vi "checkRowColor.vi"(8 "error in (no error)":errorcluster, 9 "add/delete":bool, 10 "Table in":refnum<vi>, 11 "reference in":refnum<class "Project Panels.lvclass">) -> (0 "error out":errorcluster, 3 "reference out":refnum<class "Project Panels.lvclass">)   [LabVIEW 2014, in "Project Panels.lvclass"]
uses:
  Project Panels.lvclass
  SYS/Notification Controller_class/Notification Controller.lvclass
  APP/trackingNotification_class/trackingNotification.lvclass
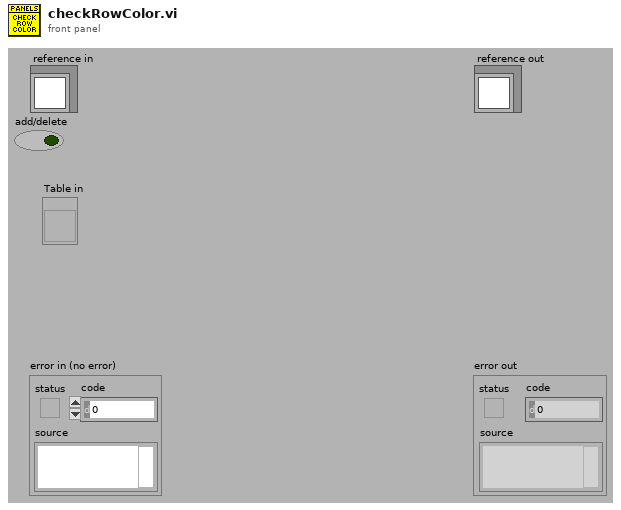
[diagram p1: front panel]
types:
  T1 = typedef "Project Panels.lvclass/ObjectAttributesRef.ctl" = refnum<data-value>
  T2 = typedef "Project Panels.lvclass/ObjectAttributes.ctl" = cluster{"MyAttribute":dbl, "device_controller_ref":refnum<class "Devices Controller.lvclass">, "file_controller_ref":refnum<class "File Controller.lvclass">, "item_controller_ref":refnum<class "Items Controller.lvclass">, "item_tables":cluster{"checkIN":string[][], "checkOUT":string[][], "storage":string[][]}, "quickbook_table":cluster{"notes":string[][]}, "notification_controller_ref":refnum<class "Notification Controller.lvclass">, "partstracking_controller_ref":refnum<class "PartsTracking Controller.lvclass">, "product_tables":cluster{"k4b2":string[][], "fitmate":string[][], "RMR":string[][], "CPET":string[][], "BP":string[][], "PP":string[][], "k5":string[][], "bb-pft":string[][]}, "rowsColour":u32[]}
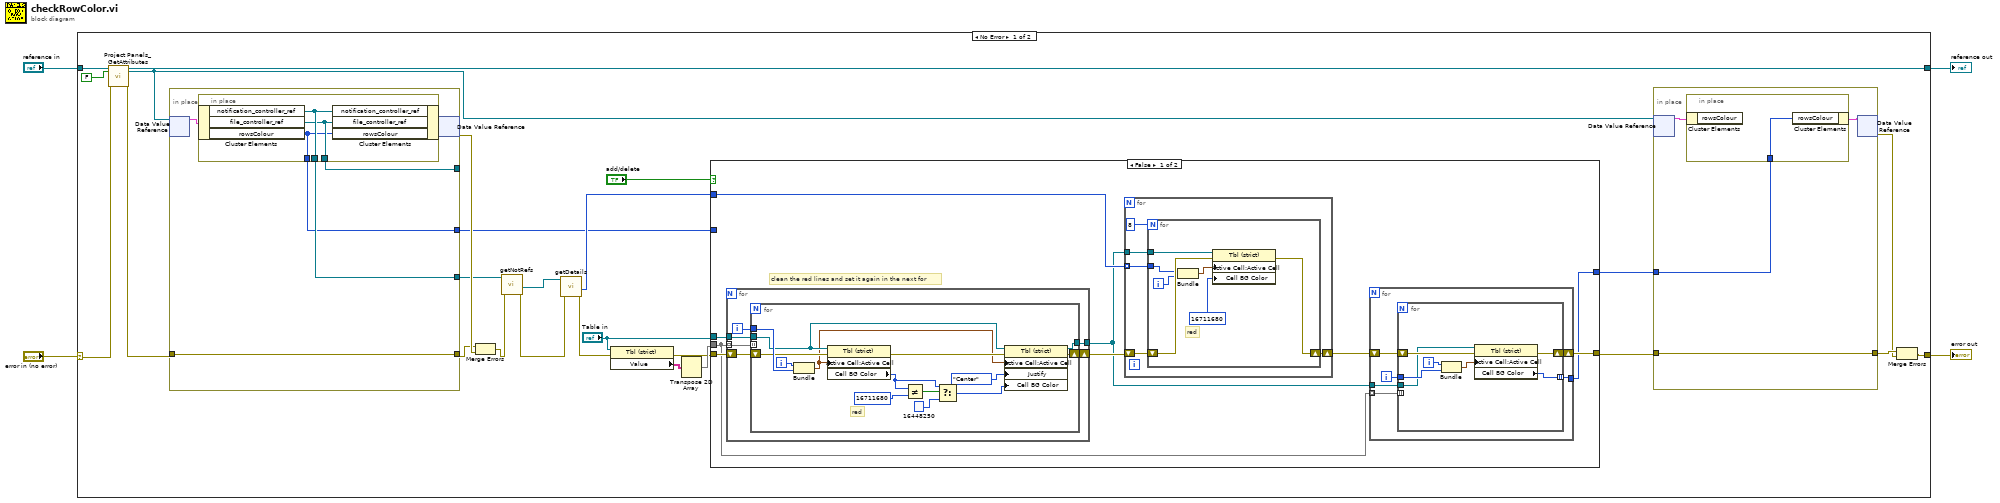
[diagram p0: block diagram]
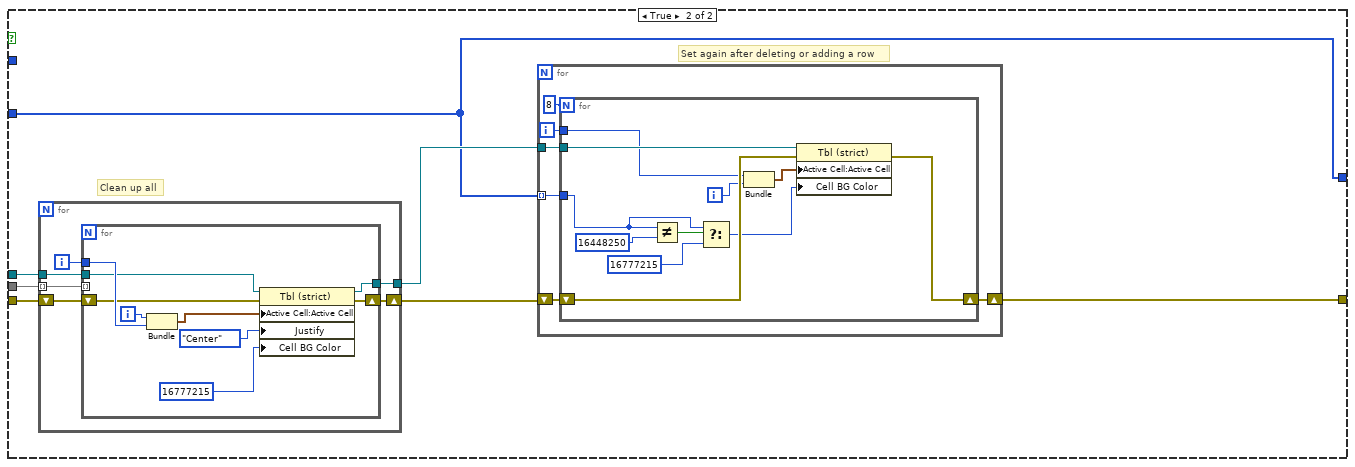
[diagram p2: hidden frame]
diagram:
  n1 = case shown="No Error" "error in (no error)" {
    selector: "error in (no error)" -> [w25 w138]
    tunnel: [w5 w138] -> w3
    tunnel: [w23 w137] -> w1
    tunnel: "reference in" -> [w27 w137]
    frame No Error {
      n2 = call "Project Panels_GetAttributes.vi"("reference in"=w27, "return data? (T)"=FALSE, "error in (no error)"=w25) -> ("reference out"=w23:refnum<class "Project Panels.lvclass">, "attributes ref"=w8:T1, "error out"=w24:errorcluster)  [unwired: 13 in, 1 out]
      n3 = in-place {
        in-place-border: w24 -> [w131]
        in-place-border: [w131] -> w28
        in-place-border: [w130] -> w19
        in-place-border: [w129] -> _
        in-place-border: [w128] -> w11
        n4 = in-place-dvr #1(w8) -> (w132:T2)  [unwired: 1 out]
        n5 = in-place {
          in-place-border: [w136] -> w130
          in-place-border: [w135] -> w129
          in-place-border: [w134] -> w128
          n6 = in-place-cluster #2(w132) -> ("notification_controller_ref"=w136:refnum<class "Notification Controller.lvclass">, "file_controller_ref"=w135:refnum<class "File Controller.lvclass">, "rowsColour"=w134:u32[])
          n7 = in-place-cluster #2("notification_controller_ref"=w136, "file_controller_ref"=w135, "rowsColour"=w134) -> (w133:T2)
        }
        n8 = in-place-dvr #1(w133) -> (w29:errorcluster)  [unwired: 1 out]
      }
      n9 = Merge Errors(w28, w29) -> (w21:errorcluster)
      n10 = call "getNotRefs.vi"("error in (no error)"=w21, "reference in"=w19) -> ("error out"=w20:errorcluster, "tracking_notification_ref"=w22:refnum<class "trackingNotification.lvclass">)  [unwired: 6 in, 2 out]
      n11 = call "getDetails.vi"("error in (no error)"=w20, "reference in"=w22) -> ("error out"=w15:errorcluster, "index_parts_expired"=w13:i32[])  [unwired: 6 in, 2 out]
      n12 = property on="Property Node" class="Tbl (strict)"(reference="Table in", error in=w15) -> (error out=w16:errorcluster, "Value"=w18:string[][])  [unwired: 1 out]
      n13 = Transpose 2D Array(2D array=w18) -> (transposed array=w17:string[][])
      n14 = case shown="False" "add/delete" {
        tunnel: w17 -> [w36 w95]
        tunnel: w16 -> [w43 w94]
        tunnel: "Table in" -> [w41 w91]
        tunnel: [w38 w90] -> w10
        tunnel: w13 -> [w40 _]
        tunnel: w11 -> [_ w89]
        tunnel: [w35 w89] -> w9
        frame False {
          # "clean the red lines and set it again in the next for"
          n15 = for {
            tunnel: w36 -> [w62] mode=indexing
            tunnel: w41 -> [w60]
            shift-right: [w58] -> w42
            shift-left: w43 -> [w59]
            tunnel: [w57] -> w37
            i -> [w61]
            n16 = for {
              tunnel: w62 -> [_] mode=indexing
              tunnel: w61 -> [w76]
              tunnel: w60 -> [w70]
              shift-right: [w72] -> w58
              shift-left: w59 -> [w74]
              tunnel: [w64] -> w57
              i -> [w75]
              # "red"
              n17 = Bundle(w75, w76) -> (w69:cluster{i32, i32})  [unwired: 1 in]
              n18 = property on="Property Node" class="Tbl (strict)"(reference=w70, error in=w74, "Active Cell:Active Cell"=w69) -> (error out=w73:errorcluster, "Cell BG Color"=w67:u32)  [unwired: 1 out]
              n19 = Not Equal?(x=w67, y=u32 16711680) -> (x != y?=w68:bool)
              n20 = Select(t=w67, s=w68, f=u32 16448250) -> (s? t:f=w66:u32)
              n21 = property on="Property Node" class="Tbl (strict)"(reference=w70, error in=w73, "Active Cell:Active Cell"=w69, "Justify"=enum16{"Left", "Center", "Right"}."Center" ("Active Cell:Cell Justification"), "Cell BG Color"=w66) -> (reference out=w64:refnum<vi>, error out=w72:errorcluster)
            }
          }
          n22 = for {
            tunnel: w40 -> [w79] mode=indexing
            tunnel: w37 -> [w78]
            shift-right: [w80] -> w39
            shift-left: w42 -> [w81]
            n23 = for {
              N: 8 -> [_]
              shift-right: [w87] -> w80
              shift-left: w81 -> [w88]
              tunnel: w79 -> [w85]
              tunnel: w78 -> [w86]
              i -> [w84]
              # "red"
              n24 = Bundle("Numeric"=w85, w84) -> (w83:cluster{"Numeric":i32, i32})  [unwired: 1 in]
              n25 = property on="Property Node" class="Tbl (strict)"(reference=w86, error in=w88, "Active Cell:Active Cell"=w83, "Cell BG Color"=u32 16711680 ("y")) -> (error out=w87:errorcluster)  [unwired: 1 out]
            }
          }
          n26 = for {
            tunnel: w36 -> [w49] mode=indexing
            tunnel: w37 -> [w47]
            shift-right: [w45] -> w38
            shift-left: w39 -> [w46]
            tunnel: [w44] -> w35
            i -> [w48]
            n27 = for {
              tunnel: w49 -> [_] mode=indexing
              tunnel: w48 -> [w56]
              tunnel: w47 -> [w53]
              shift-right: [w51] -> w45
              shift-left: w46 -> [w54]
              tunnel: [w50] -> w44 mode=indexing
              i -> [w55]
              n28 = Bundle(w55, w56) -> (w52:cluster{i32, i32})  [unwired: 1 in]
              n29 = property on="Property Node" class="Tbl (strict)"(reference=w53, error in=w54, "Active Cell:Active Cell"=w52) -> (error out=w51:errorcluster, "Cell BG Color"=w50:u32)  [unwired: 1 out]
            }
          }
        }
        frame True {
          # "Set again after deleting or adding a row"
          # "Clean up all"
          n30 = for {
            tunnel: w95 -> [w101] mode=indexing
            tunnel: w91 -> [w99]
            shift-right: [w97] -> w92
            shift-left: w94 -> [w98]
            tunnel: [w96] -> w93
            i -> [w100]
            n31 = for {
              tunnel: w101 -> [_] mode=indexing
              tunnel: w100 -> [w110]
              tunnel: w99 -> [w106]
              shift-right: [w108] -> w97
              shift-left: w98 -> [w103]
              tunnel: [w104] -> w96
              i -> [w109]
              n32 = Bundle(w109, w110) -> (w105:cluster{i32, i32})  [unwired: 1 in]
              n33 = property on="Property Node" class="Tbl (strict)"(reference=w106, error in=w103, "Active Cell:Active Cell"=w105, "Justify"=enum16{"Left", "Center", "Right"}."Center" ("Active Cell:Cell Justification"), "Cell BG Color"=u32 16777215 ("f")) -> (reference out=w104:refnum<vi>, error out=w108:errorcluster)
            }
          }
          n34 = for {
            tunnel: w93 -> [w114]
            shift-right: [w115] -> w90
            shift-left: w92 -> [w116]
            tunnel: w89 -> [w111] mode=indexing
            i -> [w112]
            n35 = for {
              N: 8 -> [_]
              shift-right: [w126] -> w115
              shift-left: w116 -> [w127]
              tunnel: w114 -> [w125]
              tunnel: w112 -> [w120]
              tunnel: w111 -> [w118]
              i -> [w124]
              n36 = Not Equal?(x=w118, y=u32 16448250) -> (x != y?=w123:bool)
              n37 = Select(t=w118, s=w123, f=u32 16777215) -> (s? t:f=w117:u32)
              n38 = Bundle(w120, w124) -> (w119:cluster{i32, i32})  [unwired: 1 in]
              n39 = property on="Property Node" class="Tbl (strict)"(reference=w125, error in=w127, "Active Cell:Active Cell"=w119, "Cell BG Color"=w117) -> (error out=w126:errorcluster)  [unwired: 1 out]
            }
          }
        }
      }
      n40 = in-place {
        in-place-border: w10 -> [w31]
        in-place-border: [w31] -> w7
        in-place-border: w9 -> [w30]
        n41 = in-place-dvr #3(w8) -> (w32:T2)  [unwired: 1 out]
        n42 = in-place {
          in-place-border: w30 -> [w34]
          n43 = in-place-cluster #4(w32) -> ()  [unwired: 1 out]
          n44 = in-place-cluster #4("rowsColour"=w34) -> (w33:T2)
        }
        n45 = in-place-dvr #3(w33) -> (w6:errorcluster)  [unwired: 1 out]
      }
      n46 = Merge Errors(w7, w6) -> (w5:errorcluster)
    }
    frame Error {
    }
  }
  "error out" <- w3
  "reference out" <- w1
